vi "Constants.vi"() -> ()   [LabVIEW 2017, in "DebugWebSerice Shared.lvlib"]
doc: "Use this Global VI to access the GUIDs assigned to the page resources of the Custom Device."
uses:
  DebugWebSerice Shared.lvlib
panel:
  in  "Tab Control":enum32{"GUIDS", "Constants", "Properties"}(tab)
  in  "pg3":string="e924be1b-f762-4191-bbce-1e4b70138d3c"
  in  "pg2":string="adf38db8-96d7-407d-abaf-661291b8caaf"
  in  "pg1":string="3d5644e6-7864-4edb-85bf-04329ae70d7a"
  in  "DebugWebSerice":string="ace36532-88b3-4511-b793-83d645ddc83a"
  in  "Compiled.Settings":string="Compiled.Settings"
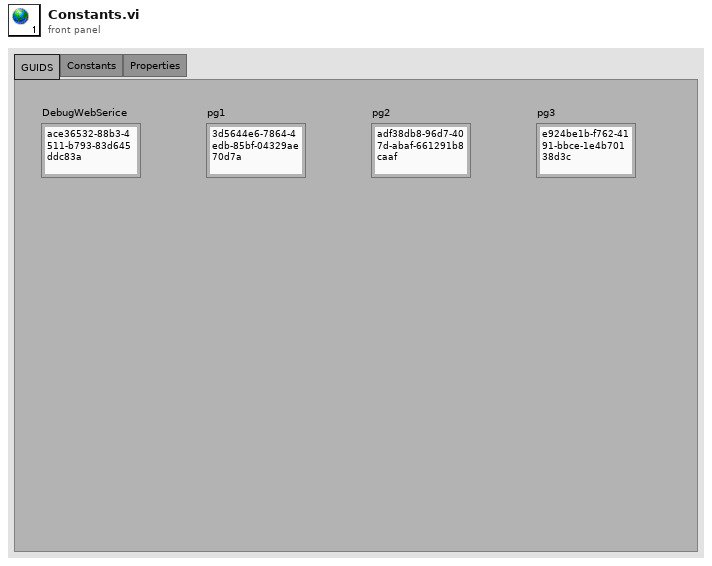
[diagram p1: front panel]
diagram:
